vi "test Subset Pointer.vi"(8 "error in (no error)":errorcluster, 11 "TestCase in":refnum<class "Lifecycle Tests.lvclass">) -> (0 "error out":errorcluster, 3 "TestCase out":refnum<class "Lifecycle Tests.lvclass">)   [LabVIEW 2020, in "Memory Manager Tests.lvlib" / "Lifecycle Tests.lvclass"]
uses:
  Lifecycle Tests.lvclass
  C:/Program Files/National Instruments/LabVIEW 2027/vi.lib/addons/_JKI Toolkits/VI Tester/TestCase.llb/TestCase.lvclass
  <vilib>/addons/_JKI Toolkits/VI Tester/TestCase.llb/TestCase.lvclass
  Classes/Pointer/Pointer.lvclass
  Classes/Pointer/Write 1D I32.vi
  Classes/Pointer/Read I32.vi
  Classes/Pointer/Write I32.vi
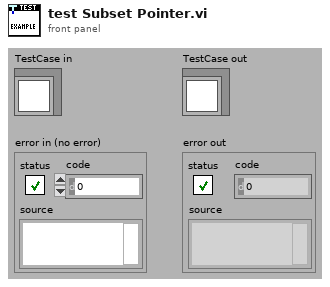
[diagram p1: front panel]
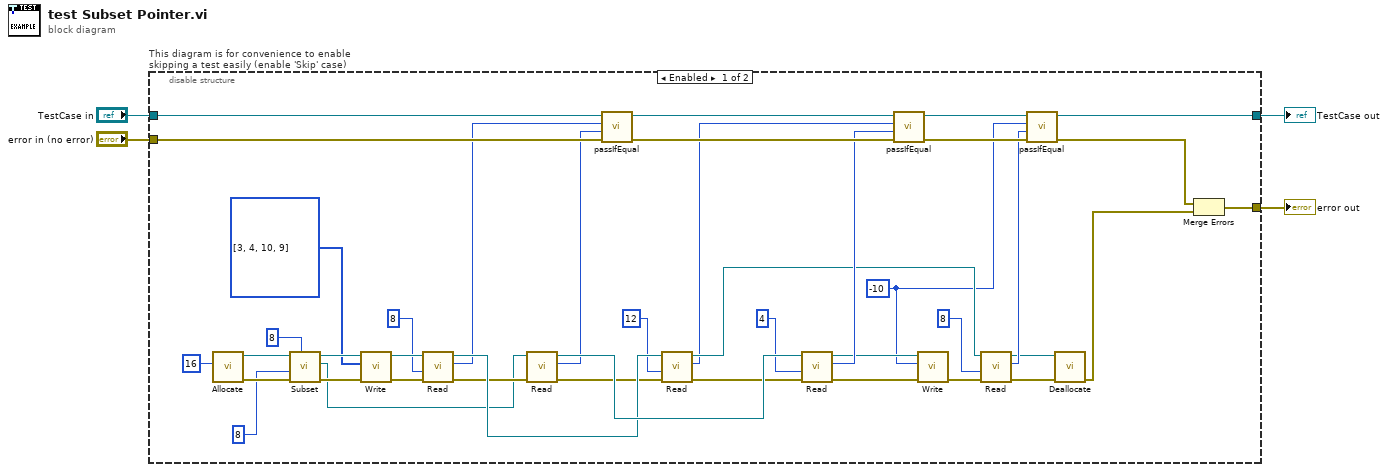
[diagram p0: block diagram]
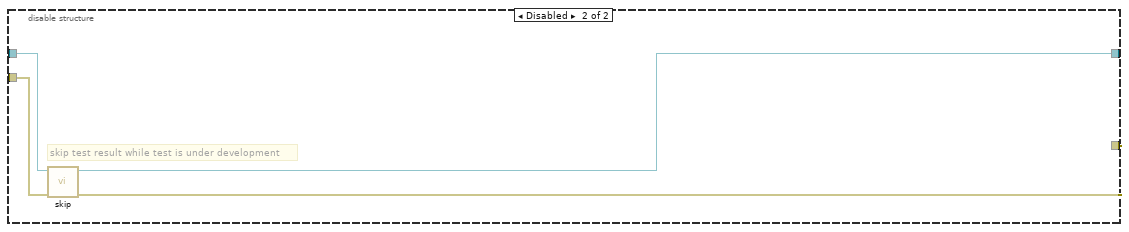
[diagram p2: hidden frame]
diagram:
  n1 = disable-structure "This diagram is for convenience to enable skipping a test easily (enable 'Skip' case)" shown="Enabled" {
    disable-tunnel: "TestCase in" -> [w30 w50]
    disable-tunnel: [w18 w48] -> w1
    disable-tunnel: [w26 w49] -> w3
    disable-tunnel: "error in (no error)" -> [w46 w47]
    frame Enabled {
      w17 = -10 ("length (-1: rest)")
      n2 = call "Allocate.vi"("size"=u64 16 ("count (1)")) -> ("error out"=w41:errorcluster, "Pointer out"=w45:refnum<class "Pointer.lvclass">)  [unwired: 9 in]
      n3 = call "Subset.vi"("length (-1: rest)"=i64 8, "error in (no error)"=w41, "offset (0)"=u64 8, "base Pointer in"=w45) -> ("error out"=w36:errorcluster, "subset Pointer"=w6:refnum<class "Pointer.lvclass">, "base Pointer out"=w43:refnum<class "Pointer.lvclass">)  [unwired: 4 in, 1 out]
      n4 = call-poly "Write.vi"("error in (no error)"=w36, "buffer in"=i32[] [3, 4, 10, 9] ("length (-1: rest)"), "Pointer in"=w43) -> ("error out"=w40:errorcluster, "Pointer out"=w42:refnum<class "Pointer.lvclass">)  [unwired: 5 in, 2 out]
      n5 = call-poly "Read.vi"("error in (no error)"=w40, "offset (0)"=u64 8, "Pointer in"=w42) -> ("error out"=w14:errorcluster, "value out"=w5:i32, "Pointer out"=w33:refnum<class "Pointer.lvclass">)  [unwired: 5 in, 1 out]
      n6 = call-poly "Read.vi"("error in (no error)"=w14, "Pointer in"=w6) -> ("error out"=w13:errorcluster, "value out"=w8:i32, "Pointer out"=w35:refnum<class "Pointer.lvclass">)  [unwired: 6 in, 1 out]
      n7 = call-dynamic "passIfEqual.vi"("error in (no error)"=w46, "y"=w8, "x"=w5, "TestCase in"=w30) -> ("error out"=w31:errorcluster, "TestCase out"=w28:refnum<class "Lifecycle Tests.lvclass">)  [unwired: 6 in]
      n8 = call-poly "Read.vi"("error in (no error)"=w13, "offset (0)"=u64 12, "Pointer in"=w33) -> ("error out"=w12:errorcluster, "value out"=w7:i32, "Pointer out"=w21:refnum<class "Pointer.lvclass">)  [unwired: 5 in, 1 out]
      n9 = call-poly "Read.vi"("error in (no error)"=w12, "offset (0)"=u64 4, "Pointer in"=w35) -> ("error out"=w25:errorcluster, "value out"=w27:i32, "Pointer out"=w23:refnum<class "Pointer.lvclass">)  [unwired: 5 in, 1 out]
      n10 = call-dynamic "passIfEqual.vi"("error in (no error)"=w31, "y"=w27, "x"=w7, "TestCase in"=w28) -> ("error out"=w29:errorcluster, "TestCase out"=w19:refnum<class "Lifecycle Tests.lvclass">)  [unwired: 6 in]
      n11 = call-poly "Write.vi"("error in (no error)"=w25, "value"=w17, "Pointer in"=w23) -> ("error out"=w24:errorcluster)  [unwired: 5 in, 3 out]
      n12 = call-poly "Read.vi"("error in (no error)"=w24, "offset (0)"=u64 8, "Pointer in"=w21) -> ("error out"=w22:errorcluster, "value out"=w15:i32, "Pointer out"=w10:refnum<class "Pointer.lvclass">)  [unwired: 5 in, 1 out]
      n13 = call-dynamic "passIfEqual.vi"("error in (no error)"=w29, "y"=w15, "x"=w17, "TestCase in"=w19) -> ("error out"=w20:errorcluster, "TestCase out"=w18:refnum<class "Lifecycle Tests.lvclass">)  [unwired: 6 in]
      n14 = call "Deallocate.vi"("error in (no error)"=w22, "Pointer"=w10) -> ("error out"=w11:errorcluster)  [unwired: 8 in, 1 out]
      n15 = Merge Errors(w20, w11) -> (w26:errorcluster)
    }
    frame Disabled {
      # "skip test result while test is under development"
      n16 = call <vilib>:"skip.vi"("error in (no error)"=w47, "TestCase in"=w50) -> ("error out"=w49:errorcluster, "TestCase out"=w48:refnum<class "Lifecycle Tests.lvclass">)  [unwired: 8 in]
    }
  }
  "error out" <- w3
  "TestCase out" <- w1
